vi "GenFile.vi"(8 "error in":errorcluster, 11 "Config":T1) -> (0 "error out":errorcluster, 3 "FileContents":string)   [LabVIEW 2017]
uses:
  <vilib>/WebServerConfig/Config.ctl
  <vilib>/WebServerConfig/Server.ctl
  <vilib>/WebServerConfig/Alias.ctl
  <vilib>/WebServerConfig/ErrorDocument.ctl
  <vilib>/WebServerConfig/Action.ctl
  <vilib>/WebServerConfig/Redirect.ctl
  <vilib>/WebServerConfig/Interface.ctl
  <vilib>/WebServerConfig/AddHandler.ctl
  <vilib>/WebServerConfig/SSL.ctl
  <vilib>/WebServerConfig/CustomLog.ctl
  <vilib>/WebServerConfig/LoadModule.ctl
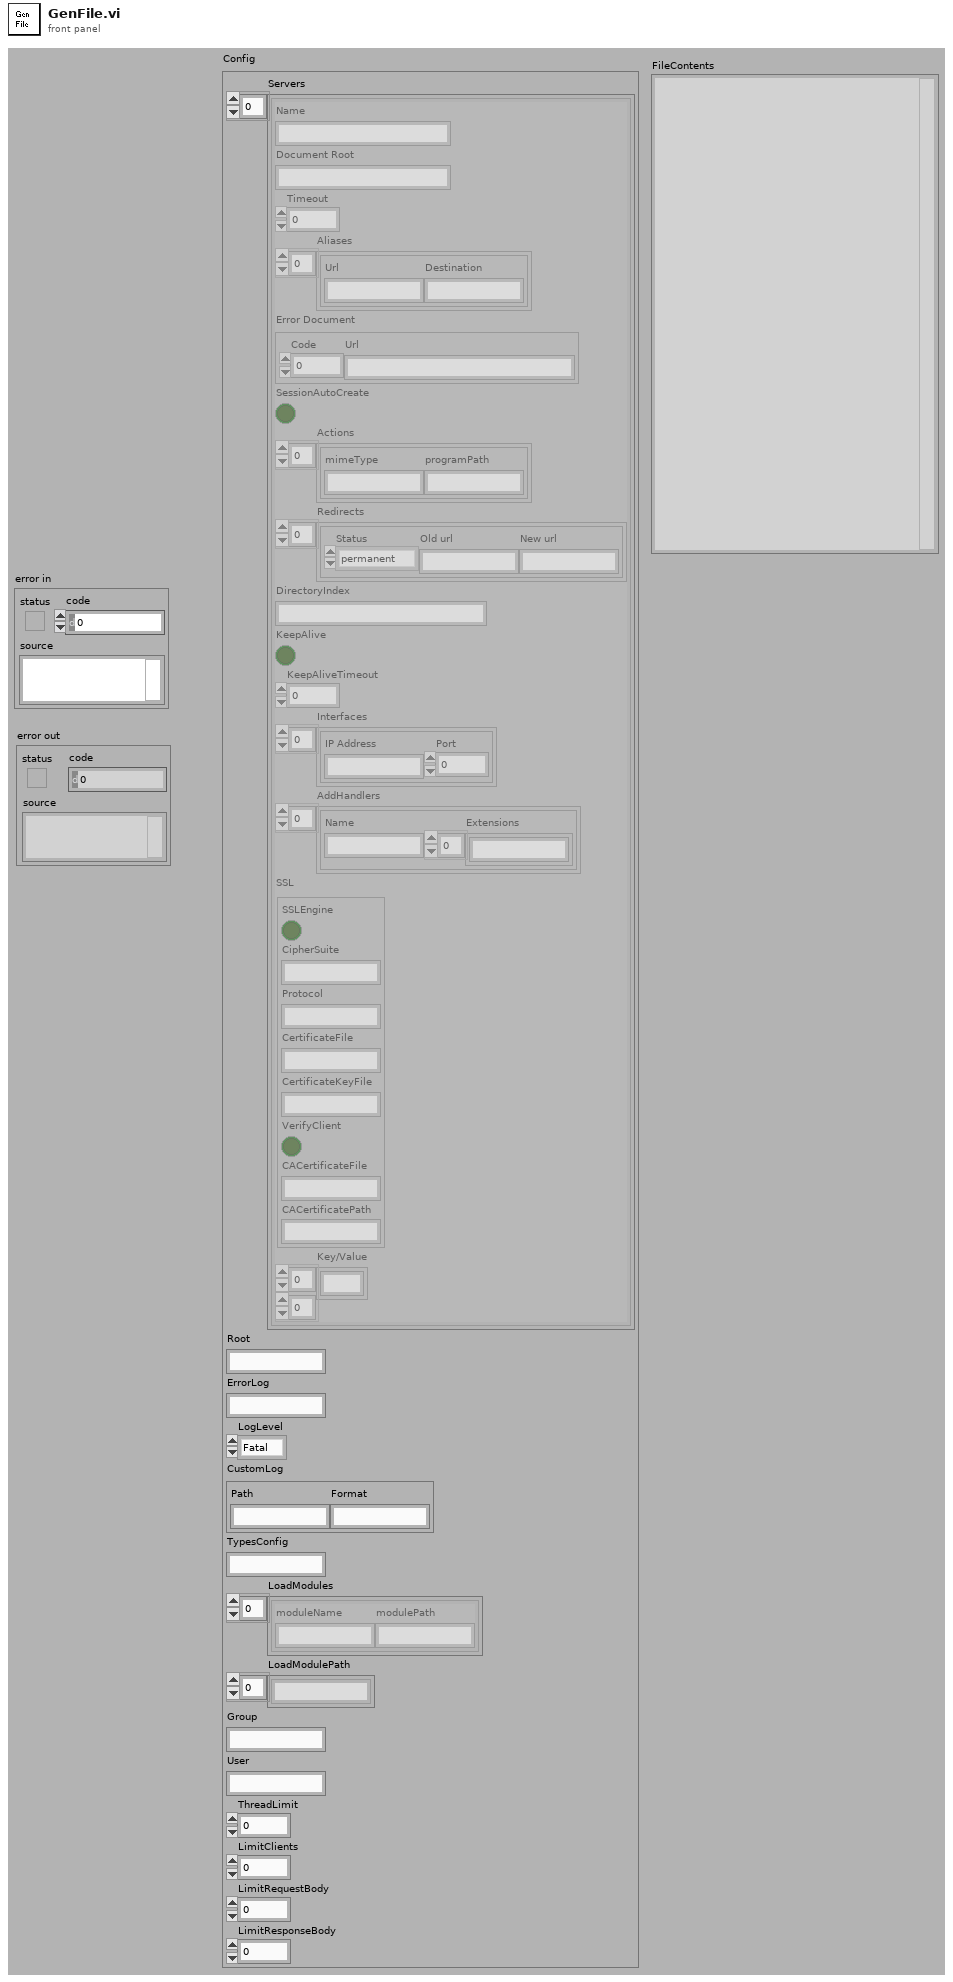
[diagram p1: front panel]
types:
  T1 = typedef "Config.ctl" = cluster{"Servers":T2[], "Root":string, "ErrorLog":string, "LogLevel":enum16{"Fatal", "Error", "Warn", "Info", "Debug", "5", "6", "7", "8", "Verbose"}, "CustomLog":T10, "TypesConfig":string, "LoadModules":T11[], "LoadModulePath":string[], "Group":string, "User":string, "ThreadLimit":u32, "LimitClients":u32, "LimitRequestBody":u32, "LimitResponseBody":u32}
  T2 = typedef "Server.ctl" = cluster{"Name":string, "Document Root":string, "Timeout":u32, "Aliases":T3[], "Error Document":T4, "SessionAutoCreate":bool, "Actions":T5[], "Redirects":T6[], "DirectoryIndex":string, "KeepAlive":bool, "KeepAliveTimeout":u32, "Interfaces":T7[], "AddHandlers":T8[], "SSL":T9, "Key/Value":string[][]}
  T3 = typedef "Alias.ctl" = cluster{"Url":string, "Destination":string}
  T4 = typedef "ErrorDocument.ctl" = cluster{"Code":u16, "Url":string}
  T5 = typedef "Action.ctl" = cluster{"mimeType":string, "programPath":string}
  T6 = typedef "Redirect.ctl" = cluster{"Status":enum16{"permanent", "temp", "seeother", "gone"}, "Old url":string, "New url":string}
  T7 = typedef "Interface.ctl" = cluster{"IP Address":string, "Port":u16}
  T8 = typedef "AddHandler.ctl" = cluster{"Name":string, "Extensions":string[]}
  T9 = typedef "SSL.ctl" = cluster{"SSLEngine":bool, "CipherSuite":string, "Protocol":string, "CertificateFile":string, "CertificateKeyFile":string, "VerifyClient":bool, "CACertificateFile":string, "CACertificatePath":string}
  T10 = typedef "CustomLog.ctl" = cluster{"Path":string, "Format":string}
  T11 = typedef "LoadModule.ctl" = cluster{"moduleName":string, "modulePath":string}
  T12 = enum16{"Global Header", "ServerRoot", "ErrorLog", "CustomLog", "TypesConfig", "Group", "User", "LimitWorkers", "LimitClients", "LimitRequestBody", "LimitResponseBody", "LoadModulePath", "LoadModules", "Listen", "DefaultServer", "VirtualServers"}
  T13 = enum16{"Fatal", "Error", "Warn", "Info", "Debug", "5", "6", "7", "8", "Verbose"}
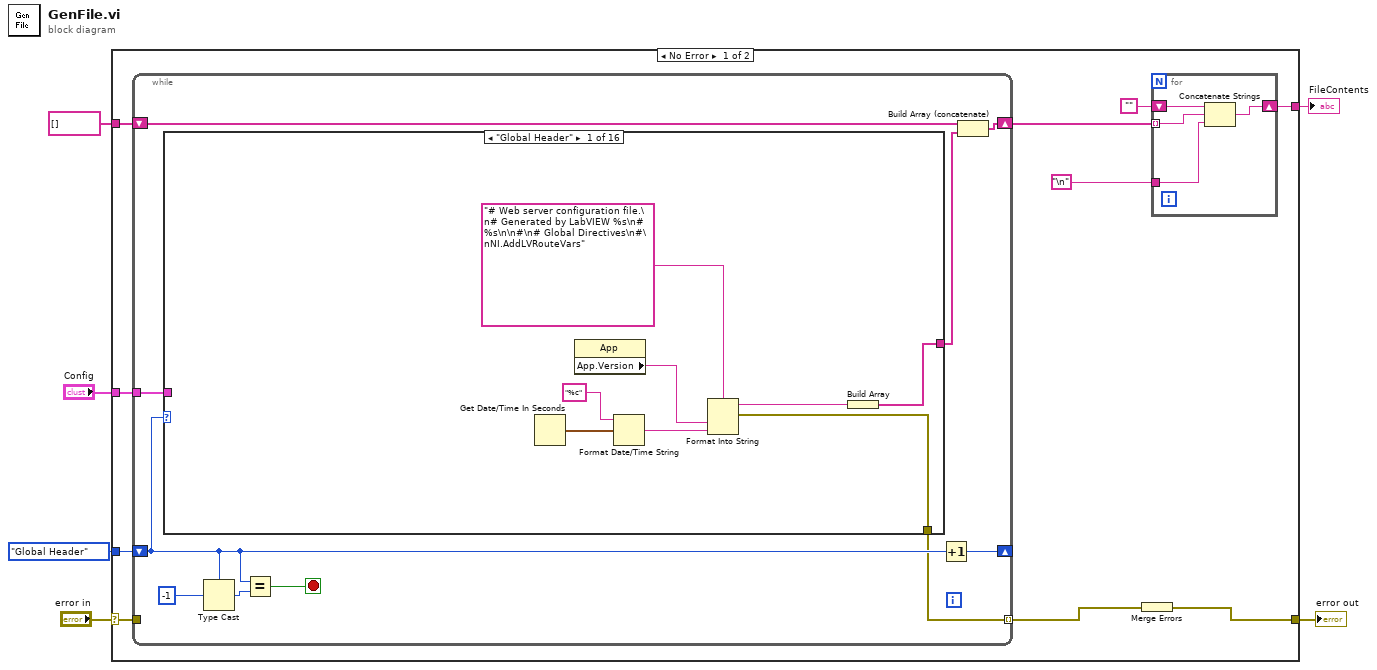
[diagram p0: block diagram]
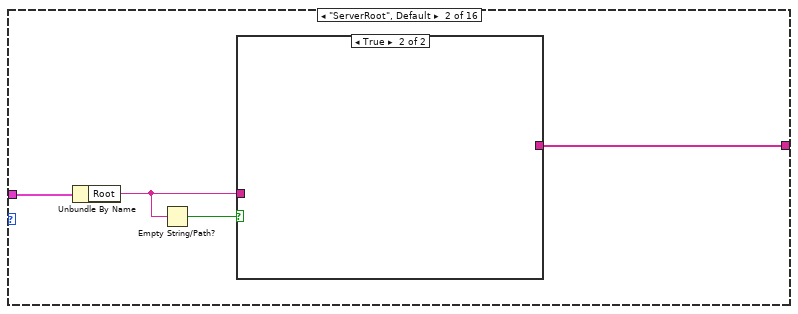
[diagram p2: hidden frame]
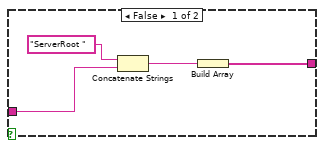
[diagram p3: hidden frame]
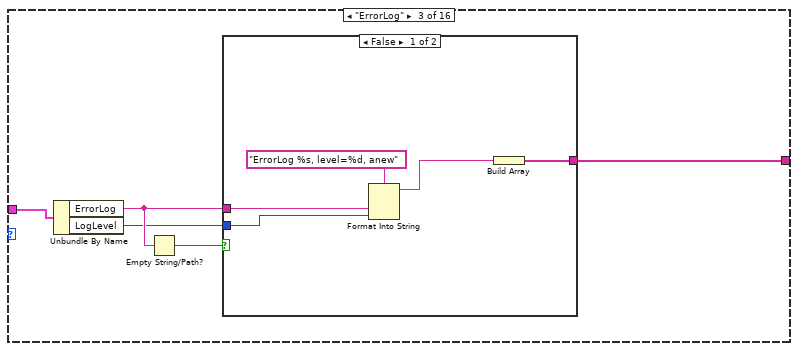
[diagram p4: hidden frame]
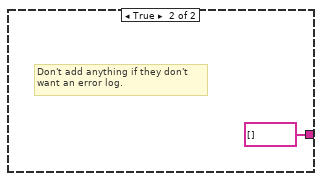
[diagram p5: hidden frame]
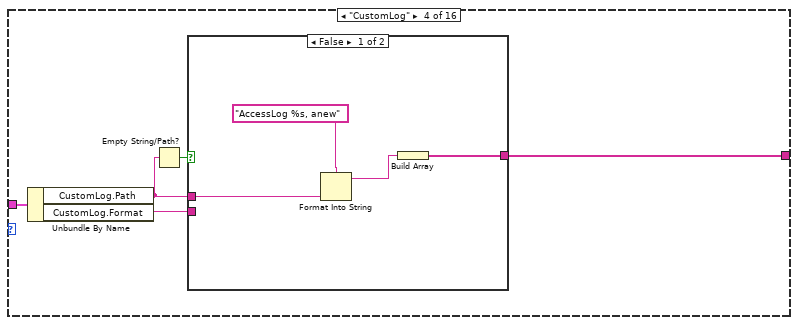
[diagram p6: hidden frame]
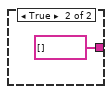
[diagram p7: hidden frame]
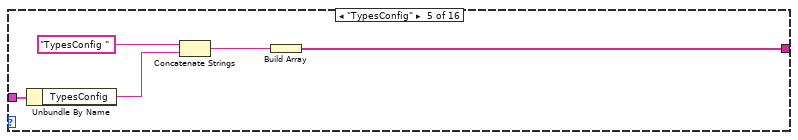
[diagram p8: hidden frame]
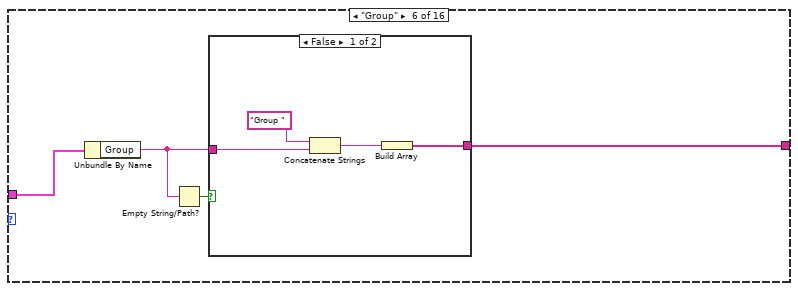
[diagram p9: hidden frame]
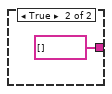
[diagram p10: hidden frame]
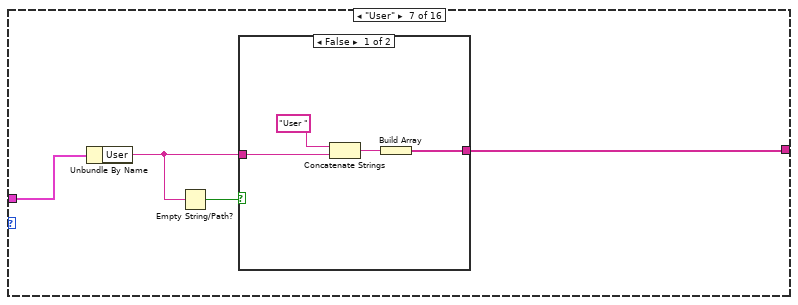
[diagram p11: hidden frame]
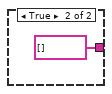
[diagram p12: hidden frame]
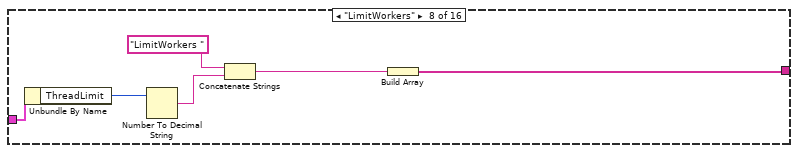
[diagram p13: hidden frame]
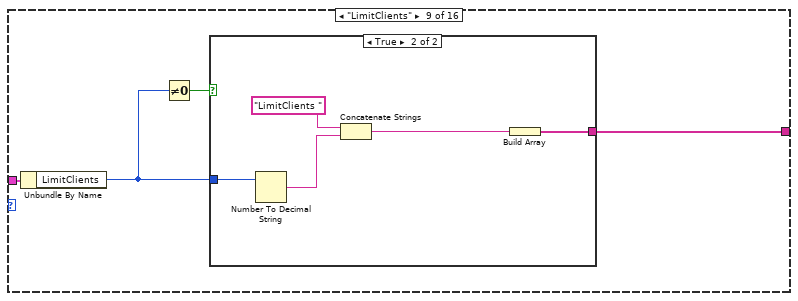
[diagram p14: hidden frame]
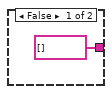
[diagram p15: hidden frame]
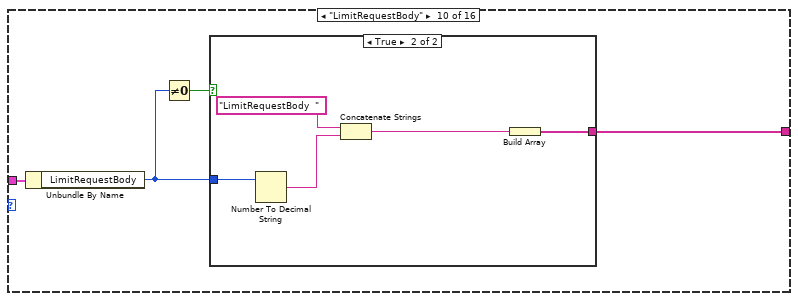
[diagram p16: hidden frame]
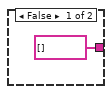
[diagram p17: hidden frame]
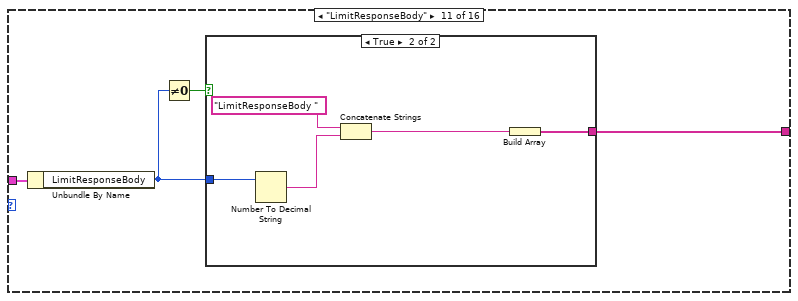
[diagram p18: hidden frame]
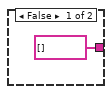
[diagram p19: hidden frame]
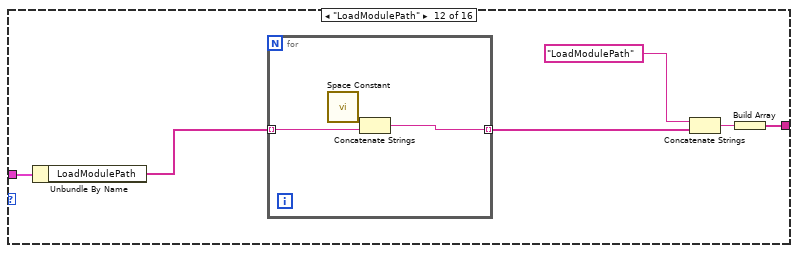
[diagram p20: hidden frame]
diagram:
  n1 = case shown="No Error" "error in" {
    selector: "error in" -> [w16 w249]
    tunnel: [w12 w249] -> w5
    tunnel: "Config" -> [w14 _]
    tunnel: T12."Global Header" -> [w15 _]
    tunnel: string[] [] -> [w13 _]
    tunnel: [w8 _] -> w1
    frame No Error {
      n2 = while {
        tunnel: w16 -> [_]
        tunnel: [w21] -> w11 mode=indexing
        shift-right: [w27] -> _
        shift-left: w15 -> [w26]
        tunnel: w14 -> [w25]
        shift-right: [w23] -> w10
        shift-left: w13 -> [w24]
        stop <- w28 stop-if-true
        n3 = case shown="\"Global Header\"" w26 {
          tunnel: w25 -> [_ w42 w51 w62 w72 w76 w85 w95 w100 w110 w120 w132 w142 w164 w202 w213]
          tunnel: [w35 w41 w50 w60 w68 w75 w84 w91 w99 w109 w119 w129 w144 w159 w198 w210] -> w22
          tunnel: [w36 _ _ _ _ _ _ _ _ _ _ _ _ _ w200 w209] -> w21
          frame "Global Header" {
            n4 = Get Date/Time In Seconds() -> (seconds since 1Jan1904=w34:timestamp)
            n5 = property class="App"() -> ("App.Version"=w31:string)  [unwired: 2 in, 2 out]
            n6 = Format Date/Time String(time format string (%c)="%c", seconds (now)=w34) -> (date/time string=w32:string)  [unwired: 1 out]
            n7 = Format Into String(format string="# Web server configuration file.\n# Generated by LabVIEW %s\n# %s\n\n#\n# Global Directives\n#\nNI.AddLVRouteVars", w31, w32) -> (resulting string=w37:string, error out=w36:errorcluster)  [unwired: 2 in]
            n8 = Build Array(w37) -> (w35:string[])
          }
          frame "ServerRoot", Default {
            n9 = Unbundle By Name(w42) -> ("Root"=w40:string)
            n10 = Empty String/Path?(string/path=w40) -> (empty?=w39:bool)
            n11 = case shown="True" w39 {
              tunnel: [w44 _] -> w41
              tunnel: w40 -> [w43 _]
              frame False {
                n12 = Concatenate Strings("ServerRoot ", w43) -> (w45:string)
                n13 = Build Array(w45) -> (w44:string[])
              }
              frame True {
              }
            }
          }
          frame "ErrorLog" {
            n14 = Unbundle By Name(w51) -> ("ErrorLog"=w49:string, "LogLevel"=w47:T13)
            n15 = Empty String/Path?(string/path=w49) -> (empty?=w48:bool)
            n16 = case shown="False" w48 {
              tunnel: [w56 string[] []] -> w50
              tunnel: w49 -> [w55 _]
              tunnel: w47 -> [w54 _]
              frame False {
                n17 = Format Into String(format string="ErrorLog %s, level=%d, anew", w55, w54) -> (resulting string=w53:string)  [unwired: 2 in, 1 out]
                n18 = Build Array(w53) -> (w56:string[])
              }
              frame True {
                # "Don't add anything if they don't\nwant an error log."
              }
            }
          }
          frame "CustomLog" {
            n19 = Unbundle By Name(w62) -> ("CustomLog.Path"=w58:string, "CustomLog.Format"=w61:string)
            n20 = Empty String/Path?(string/path=w58) -> (empty?=w59:bool)
            n21 = case shown="False" w59 {
              tunnel: w58 -> [w65 _]
              tunnel: w61 -> [_ _]
              tunnel: [w66 string[] []] -> w60
              frame False {
                n22 = Format Into String(format string="AccessLog %s, anew" ("string"), w65) -> (resulting string=w64:string)  [unwired: 2 in, 1 out]
                n23 = Build Array(w64) -> (w66:string[])
              }
              frame True {
              }
            }
          }
          frame "TypesConfig" {
            n24 = Unbundle By Name(w72) -> ("TypesConfig"=w71:string)
            n25 = Concatenate Strings("TypesConfig " ("string"), w71) -> (w70:string)
            n26 = Build Array(w70) -> (w68:string[])
          }
          frame "Group" {
            n27 = Unbundle By Name(w76) -> ("Group"=w73:string)
            n28 = Empty String/Path?(string/path=w73) -> (empty?=w74:bool)
            n29 = case shown="False" w74 {
              tunnel: w73 -> [w80 _]
              tunnel: [w77 string[] []] -> w75
              frame False {
                n30 = Concatenate Strings("Group " ("string"), w80) -> (w78:string)
                n31 = Build Array(w78) -> (w77:string[])
              }
              frame True {
              }
            }
          }
          frame "User" {
            n32 = Unbundle By Name(w85) -> ("User"=w83:string)
            n33 = Empty String/Path?(string/path=w83) -> (empty?=w82:bool)
            n34 = case shown="False" w82 {
              tunnel: w83 -> [w89 _]
              tunnel: [w86 string[] []] -> w84
              frame False {
                n35 = Concatenate Strings("User " ("string"), w89) -> (w87:string)
                n36 = Build Array(w87) -> (w86:string[])
              }
              frame True {
              }
            }
          }
          frame "LimitWorkers" {
            n37 = Unbundle By Name(w95) -> ("ThreadLimit"=w93:u32)
            n38 = Number To Decimal String(number=w93) -> (decimal integer string=w92:string)  [unwired: 1 out]
            n39 = Concatenate Strings("LimitWorkers " ("string"), w92) -> (w94:string)
            n40 = Build Array(w94) -> (w91:string[])
          }
          frame "LimitClients" {
            n41 = Unbundle By Name(w100) -> ("LimitClients"=w97:u32)
            n42 = Not Equal To 0?(x=w97) -> (x != 0?=w98:bool)
            n43 = case shown="True" w98 {
              tunnel: w97 -> [_ w105]
              tunnel: [string[] [] w102] -> w99
              frame False {
              }
              frame True {
                n44 = Number To Decimal String(number=w105) -> (decimal integer string=w104:string)  [unwired: 1 out]
                n45 = Concatenate Strings("LimitClients " ("string"), w104) -> (w103:string)
                n46 = Build Array(w103) -> (w102:string[])
              }
            }
          }
          frame "LimitRequestBody" {
            n47 = Unbundle By Name(w110) -> ("LimitRequestBody"=w107:u32)
            n48 = Not Equal To 0?(x=w107) -> (x != 0?=w108:bool)
            n49 = case shown="True" w108 {
              tunnel: w107 -> [_ w115]
              tunnel: [string[] [] w112] -> w109
              frame False {
              }
              frame True {
                n50 = Number To Decimal String(number=w115) -> (decimal integer string=w114:string)  [unwired: 1 out]
                n51 = Concatenate Strings("LimitRequestBody  " ("string"), w114) -> (w113:string)
                n52 = Build Array(w113) -> (w112:string[])
              }
            }
          }
          frame "LimitResponseBody" {
            n53 = Unbundle By Name(w120) -> ("LimitResponseBody"=w117:u32)
            n54 = Not Equal To 0?(x=w117) -> (x != 0?=w118:bool)
            n55 = case shown="True" w118 {
              tunnel: w117 -> [_ w125]
              tunnel: [string[] [] w122] -> w119
              frame False {
              }
              frame True {
                n56 = Number To Decimal String(number=w125) -> (decimal integer string=w124:string)  [unwired: 1 out]
                n57 = Concatenate Strings("LimitResponseBody " ("string"), w124) -> (w123:string)
                n58 = Build Array(w123) -> (w122:string[])
              }
            }
          }
          frame "LoadModulePath" {
            n59 = Unbundle By Name(w132) -> ("LoadModulePath"=w128:string[])
            n60 = for {
              tunnel: w128 -> [w135] mode=indexing
              tunnel: [w134] -> w127 mode=indexing
              n61 = call <vilib>:"Space Constant.vi"() -> ("String"=w133:string)
              n62 = Concatenate Strings(w133, w135) -> (w134:string)
            }
            n63 = Concatenate Strings("LoadModulePath" ("string"), w127) -> (w130:string)
            n64 = Build Array(w130) -> (w129:string[])
          }
          frame "LoadModules" {
            # "Hack alert!\nWeb services must always\nbe loaded last!"
            n65 = call <vilib>:"AddLoadModules.vi"("Config in"=w142) -> ("Config out"=w141:T1)  [unwired: 1 in, 9 out]
            n66 = Unbundle By Name(w141) -> ("LoadModules"=w138:T11[])
            n67 = call <vilib>:"FindLoadModule.vi"("Name"="WSRuntime", "LoadModules"=w138) -> ("Found"=w139:bool, "Index"=w136:i32)  [unwired: 2 in, 6 out]
            n68 = case shown="True" w139 {
              tunnel: w138 -> [w145 w150]
              tunnel: [w145 w146] -> w137
              tunnel: w136 -> [_ w149]
              frame False {
              }
              frame True {
                n69 = Delete From Array(array=w150, index=w149) -> (deleted portion=w147:T11, array with subset deleted=w148:T11[])  [unwired: 1 in]
                n70 = Build Array (concatenate)(w148, w147) -> (w146:T11[])
              }
            }
            n71 = for {
              tunnel: w137 -> [w158] mode=indexing
              shift-right: [w157] -> w144
              shift-left: string[] [] -> [w156]
              n72 = Unbundle By Name(w158) -> ("moduleName"=w155:string, "modulePath"=w154:string)
              n73 = call <vilib>:"Space Constant.vi"() -> ("String"=w151:string)
              n74 = Concatenate Strings("LoadModule " ("string"), w155, w151, w154) -> (w153:string)
              n75 = Build Array (concatenate)(w156, w153) -> (w157:string[])
            }
          }
          frame "Listen" {
            n76 = Unbundle By Name(w164) -> ("Servers"=w163:T2[])
            n77 = for {
              tunnel: w163 -> [w184] mode=indexing
              shift-right: [w181] -> w161
              shift-left: T7[] [] -> [w182]
              n78 = Unbundle By Name(w184) -> ("Interfaces"=w183:T7[])
              n79 = for {
                tunnel: w183 -> [w188] mode=indexing
                shift-right: [w187] -> w181
                shift-left: w182 -> [w185]
                n80 = call <vilib>:"FindInterfacesInterface.vi"("Interface"=w188, "Interfaces"=w185) -> ("Index"=w189:i32)  [unwired: 1 out]
                n81 = Less Than 0?(x=w189) -> (x < 0?=w186:bool)
                n82 = case shown="True" w186 {
                  tunnel: w188 -> [_ w193]
                  tunnel: [w190 w192] -> w187
                  tunnel: w185 -> [w190 w191]
                  frame False {
                  }
                  frame True {
                    n83 = Build Array (concatenate)(w191, w193) -> (w192:T7[])
                  }
                }
              }
            }
            n84 = for {
              tunnel: w161 -> [w180] mode=indexing
              shift-right: [w177] -> w159
              shift-left: string[] [] -> [w176]
              n85 = Unbundle By Name(w180) -> ("IP Address"=w169:string, "Port"=w173:u16)
              n86 = Empty String/Path?(string/path=w169) -> (empty?=w167:bool)
              n87 = Concatenate Strings(w169, ":" ("string")) -> (w165:string)
              n88 = Number To Decimal String(number=w173) -> (decimal integer string=w172:string)  [unwired: 1 out]
              n89 = Equal?(x=w169, y="*") -> (x = y?=w170:bool)
              n90 = Or(x=w167, y=w170) -> (x .or. y?=w171:bool)
              n91 = Select(t="", s=w171, f=w165) -> (s? t:f=w174:string)
              n92 = Concatenate Strings("Listen " ("string"), w174, w172) -> (w178:string)
              n93 = Build Array (concatenate)(w176, w178) -> (w177:string[])
            }
          }
          frame "DefaultServer" {
            # "Never Enable SSL for the default host"
            n94 = Unbundle By Name(w202) -> ("Servers"=w201:T2[])
            n95 = Index Array(array=w201) -> (element=w196:T2)  [unwired: 1 in]
            n96 = Bundle By Name(cluster=w196, "SSL.SSLEngine"=FALSE) -> (w195:T2)
            n97 = call <vilib>:"GenServer.vi"("Server"=w195) -> ("error out"=w200:errorcluster, "Lines"=w199:string[])  [unwired: 1 in, 8 out]
            n98 = Build Array (concatenate)("\n#\n# Directives that apply to the default server\n#", w199) -> (w198:string[])
          }
          frame "VirtualServers" {
            n99 = Unbundle By Name(w213) -> ("Servers"=w207:T2[])
            n100 = Array Subset(array=w207, index=1) -> (w212:T2[])  [unwired: 1 in]
            n101 = Index Array(array=w207) -> (element=w206:T2)  [unwired: 1 in]
            n102 = for {
              tunnel: w212 -> [w223] mode=indexing
              shift-right: [w226] -> w210
              shift-left: string[] [] -> [w224]
              tunnel: w206 -> [w222]
              tunnel: [w219] -> w205 mode=indexing
              tunnel: [w214] -> w203 mode=indexing
              n103 = Unbundle By Name(w223) -> ("Name"=w216:string, "Interfaces"=w227:T7[])
              n104 = call <vilib>:"GenServer.vi"("Default Server"=w222, "Server"=w223) -> ("error out"=w219:errorcluster, "Unique Handlers"=w221:bool, "Lines"=w220:string[])  [unwired: 1 in, 6 out]
              n105 = for {
                tunnel: w227 -> [w247] mode=indexing
                tunnel: w221 -> [w230]
                tunnel: w220 -> [w229]
                shift-right: [w236] -> w225
                shift-left: string[] [] -> [w228]
                n106 = Unbundle By Name(w247) -> ("IP Address"=w240:string, "Port"=w239:u16)
                n107 = Number To Decimal String(number=w239) -> (decimal integer string=w241:string)  [unwired: 1 out]
                n108 = Equal To 0?(x=w239) -> (x = 0?=w243:bool)
                n109 = Concatenate Strings(":", w241) -> (w244:string)
                n110 = Select(t="", s=w243, f=w244) -> (s? t:f=w238:string)
                n111 = Concatenate Strings("<VirtualHost ", w240, w238, ">") -> (w232:string)
                n112 = Build Array(w232, "Reset pipeline") -> (w233:string[])
                n113 = Build Array(w232) -> (w231:string[])
                n114 = Select(t=w233, s=w230, f=w231) -> (s? t:f=w235:string[])
                n115 = Build Array (concatenate)(w228, w235, w229, "</VirtualHost>") -> (w236:string[])
              }
              n116 = Format Into String(format string="\\n#\\n# Directives for VirtualHost %s\\n#", w216) -> (resulting string=w215:string, error out=w214:errorcluster)  [unwired: 2 in]
              n117 = Build Array (concatenate)(w224, w215, w225) -> (w226:string[])
            }
            n118 = Build Array (concatenate)(w203, w205) -> (w204:errorcluster[])
            n119 = Merge Errors(w204) -> (w209:errorcluster)
          }
        }
        n120 = Type Cast(type=w26, x=-1) -> (*(type *) &x=w29:T12)
        n121 = Equal?(x=w26, y=w29) -> (x = y?=w28:bool)
        n122 = Increment(x=w26) -> (x+1=w27:T12)
        n123 = Build Array (concatenate)(w24, w22) -> (w23:string[])
      }
      n124 = Merge Errors(w11) -> (w12:errorcluster)
      n125 = for {
        tunnel: w10 -> [w20] mode=indexing
        shift-right: [w19] -> w8
        shift-left: "" -> [w18]
        tunnel: "\n" -> [w17]
        n126 = Concatenate Strings(w18, w20, w17) -> (w19:string)
      }
    }
    frame Error {
    }
  }
  "error out" <- w5
  "FileContents" <- w1
